vi "Call_Video_Still_with_Averaging.vi"(1 "Quality":u32=750 max=1000, 2 "Resolution":T1=1 items=["Low", "Med.", "High", "Max."]) -> (0 "Error out":errorcluster)   [LabVIEW 2018]
uses:
  Camera Server/Camera enum/Camera resolution.ctl
  Anemometry Sub Vis/Globals/Meas_global.vi
  Anemometry Sub Vis/Globals/Extra_Commands_Global.vi
  Camera Server/Globals/CamServer global.vi
  Anemometry Sub Vis/Globals/Trav_pos_global.vi
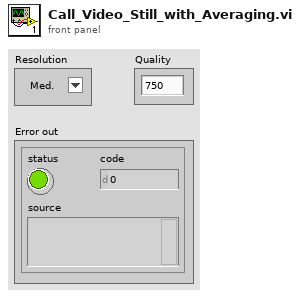
[diagram p1: front panel]
types:
  T1 = typedef "Camera resolution.ctl" = u8
  T2 = typedef "Camera enum.ctl" = string
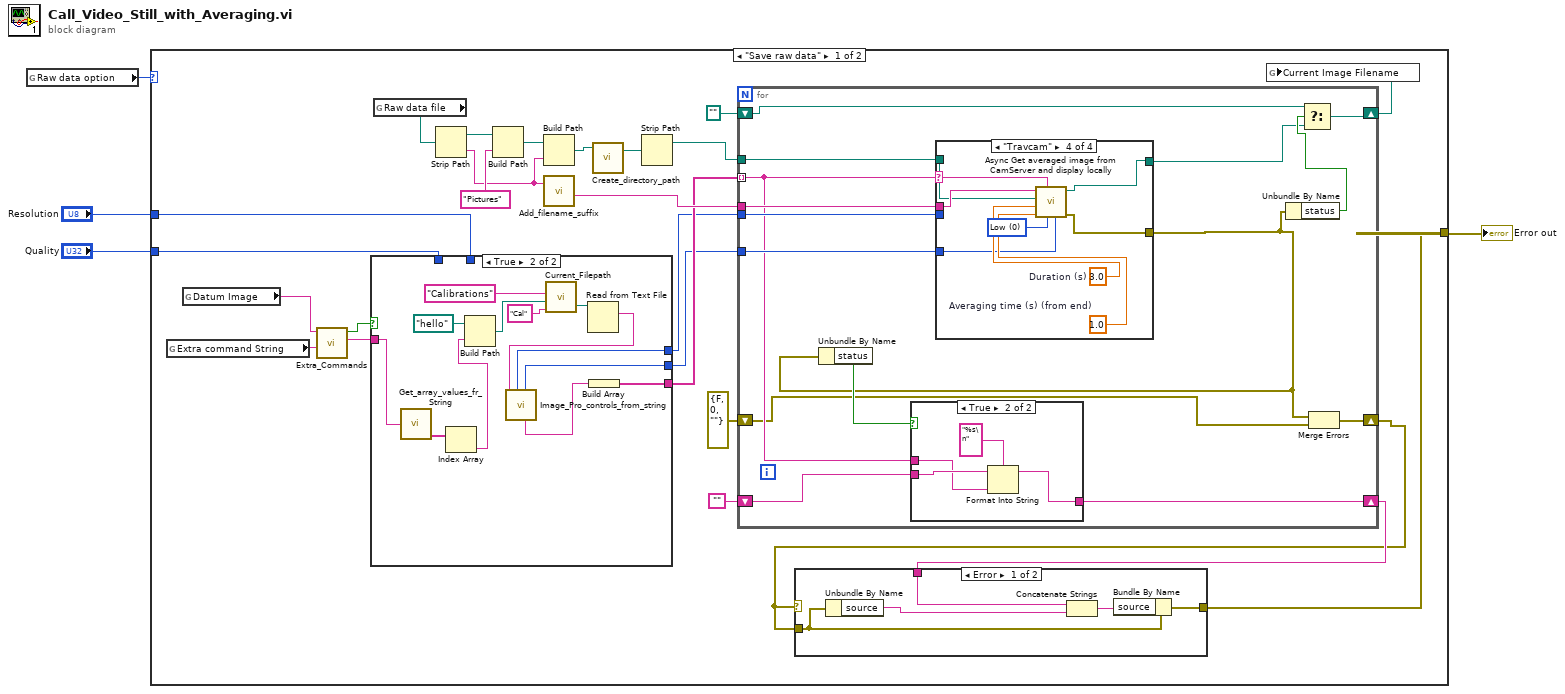
[diagram p0: block diagram]
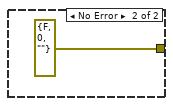
[diagram p2: hidden frame]
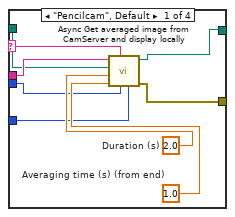
[diagram p3: hidden frame]
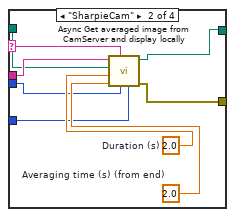
[diagram p4: hidden frame]
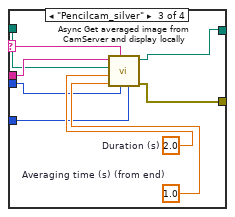
[diagram p5: hidden frame]
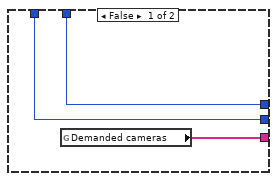
[diagram p7: hidden frame]
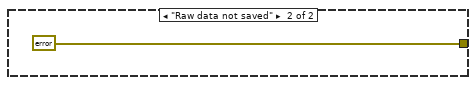
[diagram p8: hidden frame]
diagram:
  n1 = global read "Meas_global.vi" "Raw data option"() -> (w4:enum16{"Save raw data", "Raw data not saved"})
  n2 = case shown="\"Save raw data\"" w4 {
    tunnel: [w10 errorcluster {"status"=FALSE, "code"=0, "source"=""} ("Error out")] -> w3
    tunnel: "Resolution" -> [w13 _]
    tunnel: "Quality" -> [w12 _]
    frame "Save raw data" {
      n3 = global read "Meas_global.vi" "Extra command String"() -> (w16:string)
      n4 = global read "Extra_Commands_Global.vi" "Datum Image"() -> (w20:string)
      n5 = call "Extra_Commands.vi"("String to Search"=w16, "Command"=w20) -> ("String Value"=w17:string, "Command Found"=w19:bool)  [unwired: 2 in, 2 out]
      n6 = case shown="True" w19 {
        tunnel: [w94 w102] -> w18
        tunnel: w17 -> [_ w96]
        tunnel: [w92 w99] -> w15
        tunnel: [w93 w98] -> w14
        tunnel: w13 -> [w93 _]
        tunnel: w12 -> [w92 _]
        frame False {
          n7 = global read "CamServer global.vi" "Demanded cameras"() -> (w94:T2[])
        }
        frame True {
          n8 = call "Get_array_values_fr_String.vi"("String Value"=w96) -> ("String array"=w97:string[])  [unwired: 1 out]
          n9 = Index Array(array=w97) -> (element=w95:string)  [unwired: 1 in]
          n10 = Build Path(base path=path "hello", name or relative path=w95) -> (appended path=w103:path)
          n11 = call "Current_Filepath.vi"("Short_Name"="Cal" ("Data Type"), "Filename in"=w103, "Data Type"="Calibrations") -> ("Filename Out"=w107:path)  [unwired: 1 in, 1 out]
          n12 = Read from Text File(file (use dialog)=w107) -> (text=w101:string)  [unwired: 3 in, 3 out]
          n13 = call "Image_Pro_controls_from_string.vi"("Setup String"=w101) -> ("Camera"=w100:string, "Quality"=w99:u32, "Resolution"=w98:T1)  [unwired: 4 in, 4 out]
          n14 = Build Array(w100) -> (w102:string[])
        }
      }
      n15 = global read "Meas_global.vi" "Raw data file"() -> (w27:path)
      n16 = Strip Path(path=w27) -> (stripped path=w29:path, name=w23:string)
      n17 = Build Path(base path=w29, name or relative path="Pictures") -> (appended path=w26:path)
      n18 = Build Path(base path=w26, name or relative path=w23) -> (appended path=w25:path)
      n19 = call "Add_filename_suffix.vi"("Filename"=w23) -> ("Base name"=w22:string)  [unwired: 1 in, 3 out]
      n20 = call "Create_directory_path.vi"("Path name"=w25) -> ("Path name Out"=w24:path)  [unwired: 2 in, 1 out]
      n21 = Strip Path(path=w24) -> (stripped path=w21:path)  [unwired: 1 out]
      n22 = for {
        tunnel: w22 -> [w50]
        tunnel: w21 -> [w40]
        tunnel: w18 -> [w44] mode=indexing
        tunnel: w15 -> [w49]
        tunnel: w14 -> [w48]
        shift-right: [w46] -> w9
        shift-left: "" -> [w45]
        shift-right: [w41] -> w7
        shift-left: path "" -> [w42]
        shift-right: [w37] -> w5
        shift-left: errorcluster {"status"=FALSE, "code"=0, "source"=""} ("error IO") -> [w38]
        n23 = case shown="\"Travcam\"" w44 {
          selector: w44 -> [w52 w61 w70 w80]
          tunnel: w50 -> [w59 w68 w77 w86]
          tunnel: w40 -> [w58 w67 w76 w85]
          tunnel: [w51 w60 w69 w79] -> w36
          tunnel: w49 -> [w53 w62 w71 w81]
          tunnel: [w55 w64 w73 w82] -> w39
          tunnel: w48 -> [w54 w63 w72 _]
          frame "Pencilcam", Default {
            w56 = 1.0  # Averaging time (s) (from end)
            w57 = 2.0  # Duration (s)
            n24 = call "Async Get averaged image from CamServer and display locally.vi"("Quality"=w53, "Resolution"=w54, "Camera"=w52, "Averaging time (s) (from end)"=w56, "Duration (s)"=w57, "Image directory path"=w58, "Image name"=w59) -> ("Error out"=w51:errorcluster, "Image file path"=w55:path)  [unwired: 3 in]
          }
          frame "SharpieCam" {
            w65 = 2.0  # Averaging time (s) (from end)
            w66 = 2.0  # Duration (s)
            n25 = call "Async Get averaged image from CamServer and display locally.vi"("Quality"=w62, "Resolution"=w63, "Camera"=w61, "Averaging time (s) (from end)"=w65, "Duration (s)"=w66, "Image directory path"=w67, "Image name"=w68) -> ("Error out"=w60:errorcluster, "Image file path"=w64:path)  [unwired: 3 in]
          }
          frame "Pencilcam_silver" {
            w74 = 1.0  # Averaging time (s) (from end)
            w75 = 2.0  # Duration (s)
            n26 = call "Async Get averaged image from CamServer and display locally.vi"("Quality"=w71, "Resolution"=w72, "Camera"=w70, "Averaging time (s) (from end)"=w74, "Duration (s)"=w75, "Image directory path"=w76, "Image name"=w77) -> ("Error out"=w69:errorcluster, "Image file path"=w73:path)  [unwired: 3 in]
          }
          frame "Travcam" {
            w78 = T1 0 items=["Low", "Med.", "High", "Max."] ("Resolution")
            w83 = 1.0  # Averaging time (s) (from end)
            w84 = 3.0  # Duration (s)
            n27 = call "Async Get averaged image from CamServer and display locally.vi"("Quality"=w81, "Resolution"=w78, "Camera"=w80, "Averaging time (s) (from end)"=w83, "Duration (s)"=w84, "Image directory path"=w85, "Image name"=w86) -> ("Error out"=w79:errorcluster, "Image file path"=w82:path)  [unwired: 3 in]
          }
        }
        n28 = Unbundle By Name(w36) -> ("status"=w47:bool)
        n29 = case shown="True" w47 {
          tunnel: [w87 w89] -> w46
          tunnel: w45 -> [w87 w91]
          tunnel: w44 -> [_ w90]
          frame False {
          }
          frame True {
            n30 = Format Into String(format string="%s\n", initial string=w91, w90) -> (resulting string=w89:string)  [unwired: 1 in, 1 out]
          }
        }
        n31 = Unbundle By Name(w36) -> ("status"=w43:bool)
        n32 = Select(t=w42, s=w43, f=w39) -> (s? t:f=w41:path)
        n33 = Merge Errors(w36, w38) -> (w37:errorcluster)
      }
      n34 = case shown="Error" w5 {
        tunnel: [w33 errorcluster {"status"=FALSE, "code"=0, "source"=""} ("Error out")] -> w10
        tunnel: w9 -> [w32 _]
        tunnel: w5 -> [w34 _]
        frame Error {
          n35 = Unbundle By Name(w34) -> ("source"=w31:string)
          n36 = Concatenate Strings(w32, w31) -> (w30:string)
          n37 = Bundle By Name(cluster=w34, "source"=w30) -> (w33:errorcluster)
        }
        frame No Error {
        }
      }
      n38 = global write "Trav_pos_global.vi" "Current Image Filename"(w7) -> ()
    }
    frame "Raw data not saved" {
    }
  }
  "Error out" <- w3
